vi "json Parse I64 - string path.vi"(8 "error in (no error)":errorcluster, 9 "default":i64, 10 "path":string, 11 "JSON Document in":refnum<class "JSON Document.lvclass">) -> (0 "error out":errorcluster, 2 "value":i64, 3 "JSON Document out":refnum<class "JSON Document.lvclass">)   [LabVIEW 2015, in "JSON Document.lvclass"]
uses:
  JSON Document.lvclass
  JSON Document.lvclass/JSON Document.ctl
  rapidjson wrapper/rapidjson wrapper.lvlib
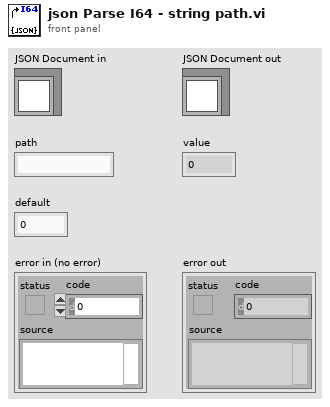
[diagram p1: front panel]
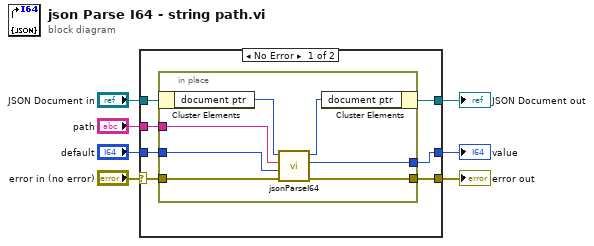
[diagram p0: block diagram]
diagram:
  n1 = case shown="No Error" "error in (no error)" {
    selector: "error in (no error)" -> [w11 w24]
    tunnel: [w10 w24] -> w6
    tunnel: [w9 w23] -> w4
    tunnel: "JSON Document in" -> [w14 w23]
    tunnel: "default" -> [w13 w22]
    tunnel: "path" -> [w12 _]
    tunnel: [w8 w22] -> w1
    frame No Error {
      n2 = in-place {
        in-place-border: w13 -> [w19]
        in-place-border: w12 -> [w18]
        in-place-border: w11 -> [w17]
        in-place-border: [w16] -> w10
        in-place-border: [w15] -> w8
        n3 = in-place-cluster #1(w14) -> ("document ptr"=w21:i64)
        n4 = call "jsonParseI64.vi"("error in (no error)"=w17, "default"=w19, "path"=w18, "d in"=w21) -> ("error out"=w16:errorcluster, "value"=w15:i64, "d out"=w20:i64)  [unwired: 5 in]
        n5 = in-place-cluster #1("document ptr"=w20) -> (w9:refnum<class "JSON Document.lvclass">)
      }
    }
    frame Error {
    }
  }
  "error out" <- w6
  "JSON Document out" <- w4
  "value" <- w1
